vi "Drive Published Globals.vi"() -> ()   [LabVIEW 2015]
doc: "This is used primarily to publish values that other subsystems or user code may want to read periodically. It may also contain some settings such as debug switches or implementation selections that are independent of the operating mode of the subsystem."
panel:
  in  "MS since drive train last moved (movement is considered 0.0001 in/s or more)":dbl
  in  "MS since drive train last moved (movement is considered .5 in/s or more)":dbl
  out "Drive Operation Finished":bool
  in  "Encoder Right":dbl
  in  "Encoder Left":dbl
  # "Tip: The global is a good way publish state or\ninformational/debugging values.\nIt is not  advised that you put setpoint values here."
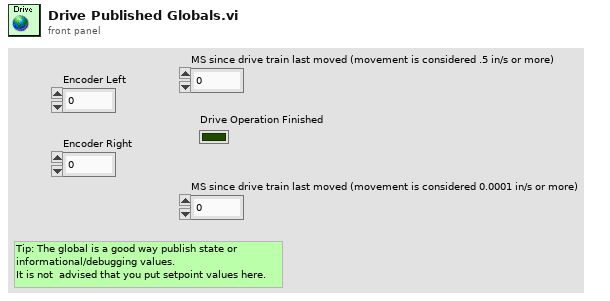
[diagram p1: front panel]
diagram:
